vi "Add VIs and their Protperties to Tree.vi"(5 "Globals?":bool=TRUE, 6 "File Extension Filters":string[](array[string]), 7 "Exclude vi.lib?":bool=TRUE, 8 "error in":errorcluster, 9 "Search Clones Up To":i32=100, 10 "AppInst":refnum<vi>, 11 "Data Tree":refnum<vi>) -> (0 "error out":errorcluster)   [LabVIEW 2013]
doc: "For a given application instance, this VI generates a tree control listing all VIs currently in memory, including all statically-referenced reentrant clones. User supplied filters are then applied. Currently active instances of any asynchronously launched reentrant VIs, which were tagged for inclusion, are also added to the tree. This tagging is accomplished by dropping the \"Clone VIs FG\" DropIn VI onto the block diagram of any reentrant VI which you wish to monitor. These tagged items will not be filtered."
uses:
  Clone VIs FG Enum.ctl
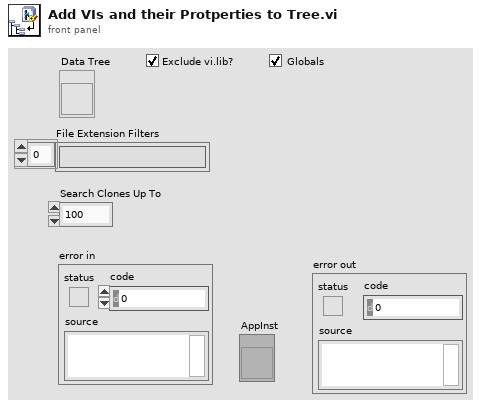
[diagram p1: front panel]
types:
  T1 = typedef "Clone VIs FG Enum.ctl" = enum16{"Get", "Get Active VIs", "Add Calling VI"}
  T2 = enum32{"invalid VI type", "Standard VI", "Control VI", "Global VI", "Polymorphic VI", "Configuration VI", "SubSystem", "Facade VI", "Method VI", "Statechart Diagram VI"}
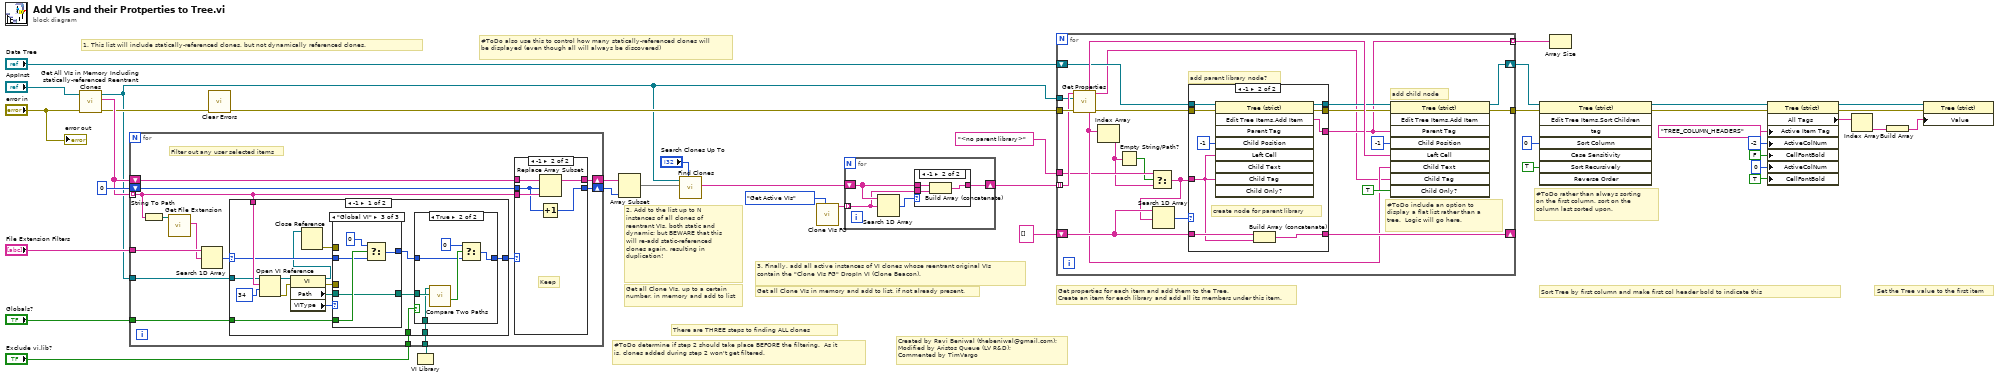
[diagram p0: block diagram]
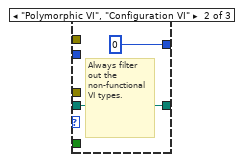
[diagram p5: hidden frame]
diagram:
  # "#ToDo also use this to control how many statically-referenced clones will be displayed (even though all will always be discovered)"
  # "#ToDo determine if step 2 should take place BEFORE the filtering.  As it is, clones added during step 2 won't get filtered."
  # "2. Add to the list up to N instances of all clones of reentrant VIs, both static and dynamic; but BEWARE that this will re-add static-referenced clones again, resulting in duplication!"
  # "Get all Clone VIs, up to a certain \nnumber, in memory and add to list"
  # "#ToDo rather than always sorting on the first column, sort on the column last sorted upon."
  # "1. This list will include statically-referenced clones, but not dynamically referenced clones."
  # "There are THREE steps to finding ALL clones"
  # "3. Finally, add all active instances of VI clones whose reentrant original VIs contain the \"Clone VIs FG\" DropIn VI (Clone Beacon)."
  # "Get all Clone VIs in memory and add to list, if not already present."
  # "Sort Tree by first column and make first col header bold to indicate this"
  # "Created by Ravi Beniwal (thebeniwal@gmail.com);\nModified by Aristos Queue (LV R&D);\nCommented by TimVargo"
  # "Set the Tree value to the first item"
  # "Get properties for each item and add them to the Tree.\nCreate an item for each library and add all its members under this item."
  n1 = call "Get All VIs in Memory Including statically-referenced Reentrant Clones.vi"("error in (no error)"="error in", "App Refnum"="AppInst") -> ("error out"=w13:errorcluster, "All VIs in Memory Including Reentrant Clones"=w15:string[], "App Refnum Out"=w1:refnum<vi>)  [unwired: 5 in, 2 out]
  n2 = call <vilib>:"Clear Errors.vi"("error in (no error)"=w13) -> ("error out"=w7:errorcluster)  [unwired: 6 in]
  n3 = VI Library() -> (path=w17:path)
  n4 = for {
    tunnel: w15 -> [w44] mode=indexing
    tunnel: "File Extension Filters" -> [w52]
    shift-right: [w49] -> w36
    shift-left: w15 -> [w50]
    shift-right: [w47] -> w35
    shift-left: 0 -> [w48]
    tunnel: "Globals?" -> [w43]
    tunnel: "Exclude vi.lib?" -> [w42]
    tunnel: w17 -> [w41]
    tunnel: w1 -> [w40]
    # "Filter out any user selected items"
    n5 = String To Path(string=w44) -> (path=w53:path)
    n6 = call <vilib>:"Get File Extension.vi"("file"=w53) -> ("lowercase file extension"=w51:string)  [unwired: 7 in, 3 out]
    n7 = Search 1D Array(1D array=w52, element=w51) -> (index of element=w46:i32)  [unwired: 1 in]
    n8 = case shown="-1" w46 {
      selector: w46 -> [w67 w87]
      tunnel: [w60 w87] -> w45
      tunnel: w44 -> [w70 _]
      tunnel: w43 -> [w65 _]
      tunnel: w42 -> [w64 _]
      tunnel: w41 -> [w62 _]
      tunnel: w40 -> [w55 _]
      frame -1 {
        n9 = Open VI Reference(application reference (local)=w55, vi path=w70, options=34) -> (vi reference=w69:refnum<vi>, error out=w58:errorcluster)  [unwired: 3 in]
        n10 = property class="VI"(reference=w69, error in=w58) -> (reference out=w59:refnum<vi>, error out=w57:errorcluster, "Path"=w66:path, "VIType"=w68:T2)
        n11 = Close Reference(reference=w59) -> (error out=w56:errorcluster)  [unwired: 1 in]
        n12 = case shown="\"Global VI\"" w68 {
          tunnel: w67 -> [w79 _ w85]
          tunnel: [w79 0 ("index of element") w84] -> w61
          tunnel: w66 -> [w78 w80 w82]
          tunnel: w65 -> [_ _ w86]
          tunnel: [w78 w80 w82] -> w63
          tunnel: w57 -> [_ _ _]
          tunnel: w56 -> [_ _ _]
          frame Default {
            # "Don't exclude"
          }
          frame "Polymorphic VI", "Configuration VI" {
            # "Always filter out the non-functional VI types."
          }
          frame "Global VI" {
            n13 = Select(t=0, s=w86, f=w85) -> (s? t:f=w84:i32)
          }
        }
        n14 = case shown="True" w64 {
          tunnel: w63 -> [_ w77]
          tunnel: w62 -> [_ w76]
          tunnel: w61 -> [w71 w74]
          tunnel: [w71 w72] -> w60
          frame False {
            # "Don't exclude items in vi.lib"
          }
          frame True {
            n15 = call <vilib>:"Compare Two Paths.vi"("Path 2"=w77, "Path 1"=w76) -> ("Path 2 Relative to Path 1?"=w75:bool)  [unwired: 6 in, 3 out]
            n16 = Select(t=0, s=w75, f=w74) -> (s? t:f=w72:i32)
          }
        }
      }
      frame Default {
      }
    }
    n17 = case shown="-1" w45 {
      tunnel: w50 -> [w89 w94]
      tunnel: [w89 w93] -> w49
      tunnel: w44 -> [_ w92]
      tunnel: w48 -> [w88 w91]
      tunnel: [w88 w90] -> w47
      frame 0, Default {
        # "Discard"
      }
      frame -1 {
        # "Keep"
        n18 = Replace Array Subset(array=w94, new element=w92, index=w91) -> (w93:string[])
        n19 = Increment(x=w91) -> (x+1=w90:i32)
      }
    }
  }
  n20 = Array Subset(array=w36, length=w35) -> (w16:string[])  [unwired: 1 in]
  n21 = call "Find Clones.vi"("Search Clones Up To"="Search Clones Up To", "VIs in"=w16, "Application in"=w1) -> ("VIs (including clones) out"=w9:string[])  [unwired: 8 in]
  n22 = call "Clone VIs FG.vi"("Action"=Clone_VIs_FG_Enum."Get Active VIs") -> ("VIs"=w10:string[])  [unwired: 9 in, 1 out]
  n23 = for {
    shift-right: [w97] -> w8
    shift-left: w9 -> [w98]
    tunnel: w10 -> [w96] mode=indexing
    n24 = Search 1D Array(1D array=w98, element=w96) -> (index of element=w95:i32)  [unwired: 1 in]
    n25 = case shown="-1" w95 {
      tunnel: w98 -> [w99 w102]
      tunnel: [w99 w101] -> w97
      tunnel: w96 -> [_ w100]
      frame 0, Default {
      }
      frame -1 {
        n26 = Build Array (concatenate)(w102, w100) -> (w101:string[])
      }
    }
  }
  n27 = for {
    tunnel: w8 -> [w120] mode=indexing
    tunnel: w7 -> [w123]
    tunnel: [w122] -> w32
    shift-right: [w121] -> w29
    shift-left: "Data Tree" -> [w113]
    tunnel: w1 -> [w118]
    shift-right: [w114] -> _
    shift-left: string[] [] -> [w115]
    tunnel: [w110] -> w4 mode=indexing
    tunnel: "<no parent library>" -> [w105]
    # "#ToDo include an option to display a flat list rather than a tree.  Logic will go here."
    # "add child node"
    # "add parent library node?"
    n28 = call "Get Properties.vi"("VI Name"=w120, "AppInst"=w118, "error in"=w123) -> ("File Name Out"=w119:string, "Full Name Out"=w107:string, "VI Properties (All)"=w108:string[], "error out"=w116:errorcluster)  [unwired: 5 in, 4 out]
    n29 = Index Array(array=w108) -> (element=w103:string)  [unwired: 1 in]
    n30 = Empty String/Path?(string/path=w103) -> (empty?=w104:bool)
    n31 = Select(t=w105, s=w104, f=w103) -> (s? t:f=w106:string)
    n32 = Search 1D Array(1D array=w115, element=w106) -> (index of element=w109:i32)  [unwired: 1 in]
    n33 = case shown="-1" w109 {
      tunnel: [w127 w136] -> w117
      tunnel: w116 -> [w127 w135]
      tunnel: [w126 w134] -> w114
      tunnel: w115 -> [w126 w133]
      tunnel: w106 -> [w125 w129]
      tunnel: w113 -> [w128 w132]
      tunnel: [w128 w131] -> w112
      tunnel: [w125 w130] -> w110
      frame 0, Default {
        # "parent library already exists"
      }
      frame -1 {
        # "create node for parent library"
        n34 = invoke on="Invoke Node" class="Tree (strict)" method="Edit Tree Items.Add Item"(reference=w132, error in=w135, "Child Position"=-1, "Left Cell"=w129, "Child Tag"=w129) -> (reference out=w131:refnum<vi>, error out=w136:errorcluster, "Edit Tree Items:Add Item"=w130:string)  [unwired: 4 in, 6 out]
        n35 = Build Array (concatenate)(w133, w129) -> (w134:string[])
      }
    }
    n36 = invoke on="Invoke Node" class="Tree (strict)" method="Edit Tree Items.Add Item"(reference=w112, error in=w117, "Parent Tag"=w110, "Child Position"=-1, "Left Cell"=w119, "Child Text"=w108, "Child Tag"=w107, "Child Only?"=TRUE) -> (reference out=w121:refnum<vi>, error out=w122:errorcluster)  [unwired: 1 in, 7 out]
  }
  n37 = invoke on="Invoke Node" class="Tree (strict)" method="Edit Tree Items.Sort Children"(reference=w29, error in=w32, "Sort Column"=0, "Sort Recursively"=TRUE ("Sort Recursively?")) -> (reference out=w30:refnum<vi>, error out=w31:errorcluster)  [unwired: 4 in, 6 out]
  n38 = Array Size(array=w4) -> ()  [unwired: 1 out]
  n39 = property class="Tree (strict)"(reference=w30, error in=w31, "Active Item Tag"="TREE_COLUMN_HEADERS" ("Active Item:Tag"), "ActiveColNum"=-2 ("Active Cell:Active Column Number"), "CellFontBold"=FALSE ("Active Cell:Cell Font:Bold"), "ActiveColNum"=0 ("Active Cell:Active Column Number"), "CellFontBold"=TRUE ("Active Cell:Cell Font:Bold")) -> (reference out=w26:refnum<vi>, error out=w27:errorcluster, "All Tags"=w28:string[])
  n40 = Index Array(array=w28) -> (element=w25:string)  [unwired: 1 in]
  n41 = Build Array(w25) -> (w34:string[])
  n42 = property class="Tree (strict)"(reference=w26, error in=w27, "Value"=w34) -> ()  [unwired: 2 out]
  "error out" <- "error in"
